vi "Create Time Array.vi"(10 "Iterations/Second":i32=10, 11 "Actual Rate":dbl) -> (1 "Time Increment":dbl, 2 "Base Time Array":dbl[](array[numeric]), 3 "Samples / Iteration":i32)   [LabVIEW 2019]
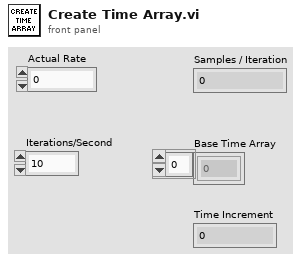
[diagram p1: front panel]
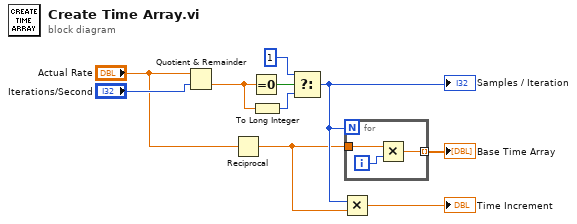
[diagram p0: block diagram]
diagram:
  n1 = Quotient & Remainder(x="Actual Rate", y="Iterations/Second") -> (floor(x/y)=w9:dbl)  [unwired: 1 out]
  n2 = Reciprocal(x="Actual Rate") -> (1/x=w1:dbl)
  n3 = Equal To 0?(x=w9) -> (x = 0?=w7:bool)
  n4 = To Long Integer(number=w9) -> (32bit integer=w10:i32)
  n5 = Select(t=1, s=w7, f=w10) -> (s? t:f=w3:i32)
  "Samples / Iteration" <- w3
  n6 = Multiply(x=w3, y=w1) -> (x*y=→"Time Increment":dbl)
  n7 = for {
    N: w3 -> [_]
    tunnel: w1 -> [w13]
    tunnel: [w11] -> w5 mode=indexing
    i -> [w12]
    n8 = Multiply(x=w13, y=w12) -> (x*y=w11:dbl)
  }
  "Base Time Array" <- w5
